vi "DriveGetDist.vi"() -> (3 "ModuleTravelPosition":dbl[](array[numeric]))   [LabVIEW 2023]
doc: "Gets left and right distance variables for drive (incorrect)\noutputs:\n--ModuleTravelPosition--array--"
uses:
  DriveGlobal.vi
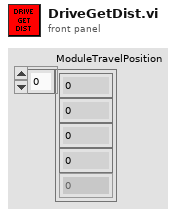
[diagram p1: front panel]
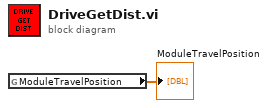
[diagram p0: block diagram]
diagram:
  n1 = global read "DriveGlobal.vi" "ModuleTravelPosition"() -> (→"ModuleTravelPosition":dbl[])
